vi "myRIO_BRig_Host_v0,35.vi"() -> ()   [LabVIEW 2014]
panel:
  in  "Pause":bool
  out "graph_ai1 2":dbl(graph)
  out "graph_ai0 2":dbl[](graph)
  out "graph_ai1":dbl(graph)
  out "RunTime_seconds":u16
  out "RunTime_minutes":u16
  out "BlockL_T2R_cur":u16 caption="Trials2Reward"
  out "BlockL_BTPR_cur":u16 caption="BadTrialsPostReward"
  out "BlockL_T2R_avg":dbl caption="Trials2Reward" format="%#_3g"
  out "BlockL_BTPR_avg":dbl caption="BadTrialsPostReward" format="%#_3g"
  out "BlockR_T2R_cur":u16 caption="Trials2Reward"
  out "BlockR_BTPR_cur":u16 caption="BadTrialsPostReward"
  out "BlockR_T2R_avg":dbl caption="Trials2Reward" format="%#_3g"
  out "BlockR_BTPR_avg":dbl caption="BadTrialsPostReward" format="%#_3g"
  out "error_LoadPrevSettings":errorcluster caption="error out"
  in  "LoadPrevSettings":bool
  out "graph_ai0":dbl(graph)
  in  "maxTrialsDisplayed":i32 caption="Number of Trials Displayed\n( 0 = all trials )"
  out "error_TCP":errorcluster
  in  "stop":bool
  in  "colorIn_timeout":u32(colorbox)=7468543 caption="Choice Timeout"
  in  "colorIn_wrong/cue":u32(colorbox)=16728618 caption="Wrong Choice or\nLicked During Cue"
  in  "colorIn_reward":u32(colorbox)=5898088 caption="Reward"
  in  "colorIn_unknown":u32(colorbox)=16449331 caption="Unknown Trial Status"
  out "dataOut_plot":cluster{i32[], i32[]}[](graph)
  out "iTrial":i32
  out "iBlock":i32
  # "Exp Stats"
  # "Current Block Stats"
  # "Trials 2 Reward\n\nBad Trials\nPost Reward"
  # "Left Spout    Right Spout"
  # "Run Time\n\n   minutes    seconds"
  # "Average Block Stats"
  # "Trials 2 Reward\n\nBad Trials\nPost Reward"
  # "Left Spout    Right Spout"
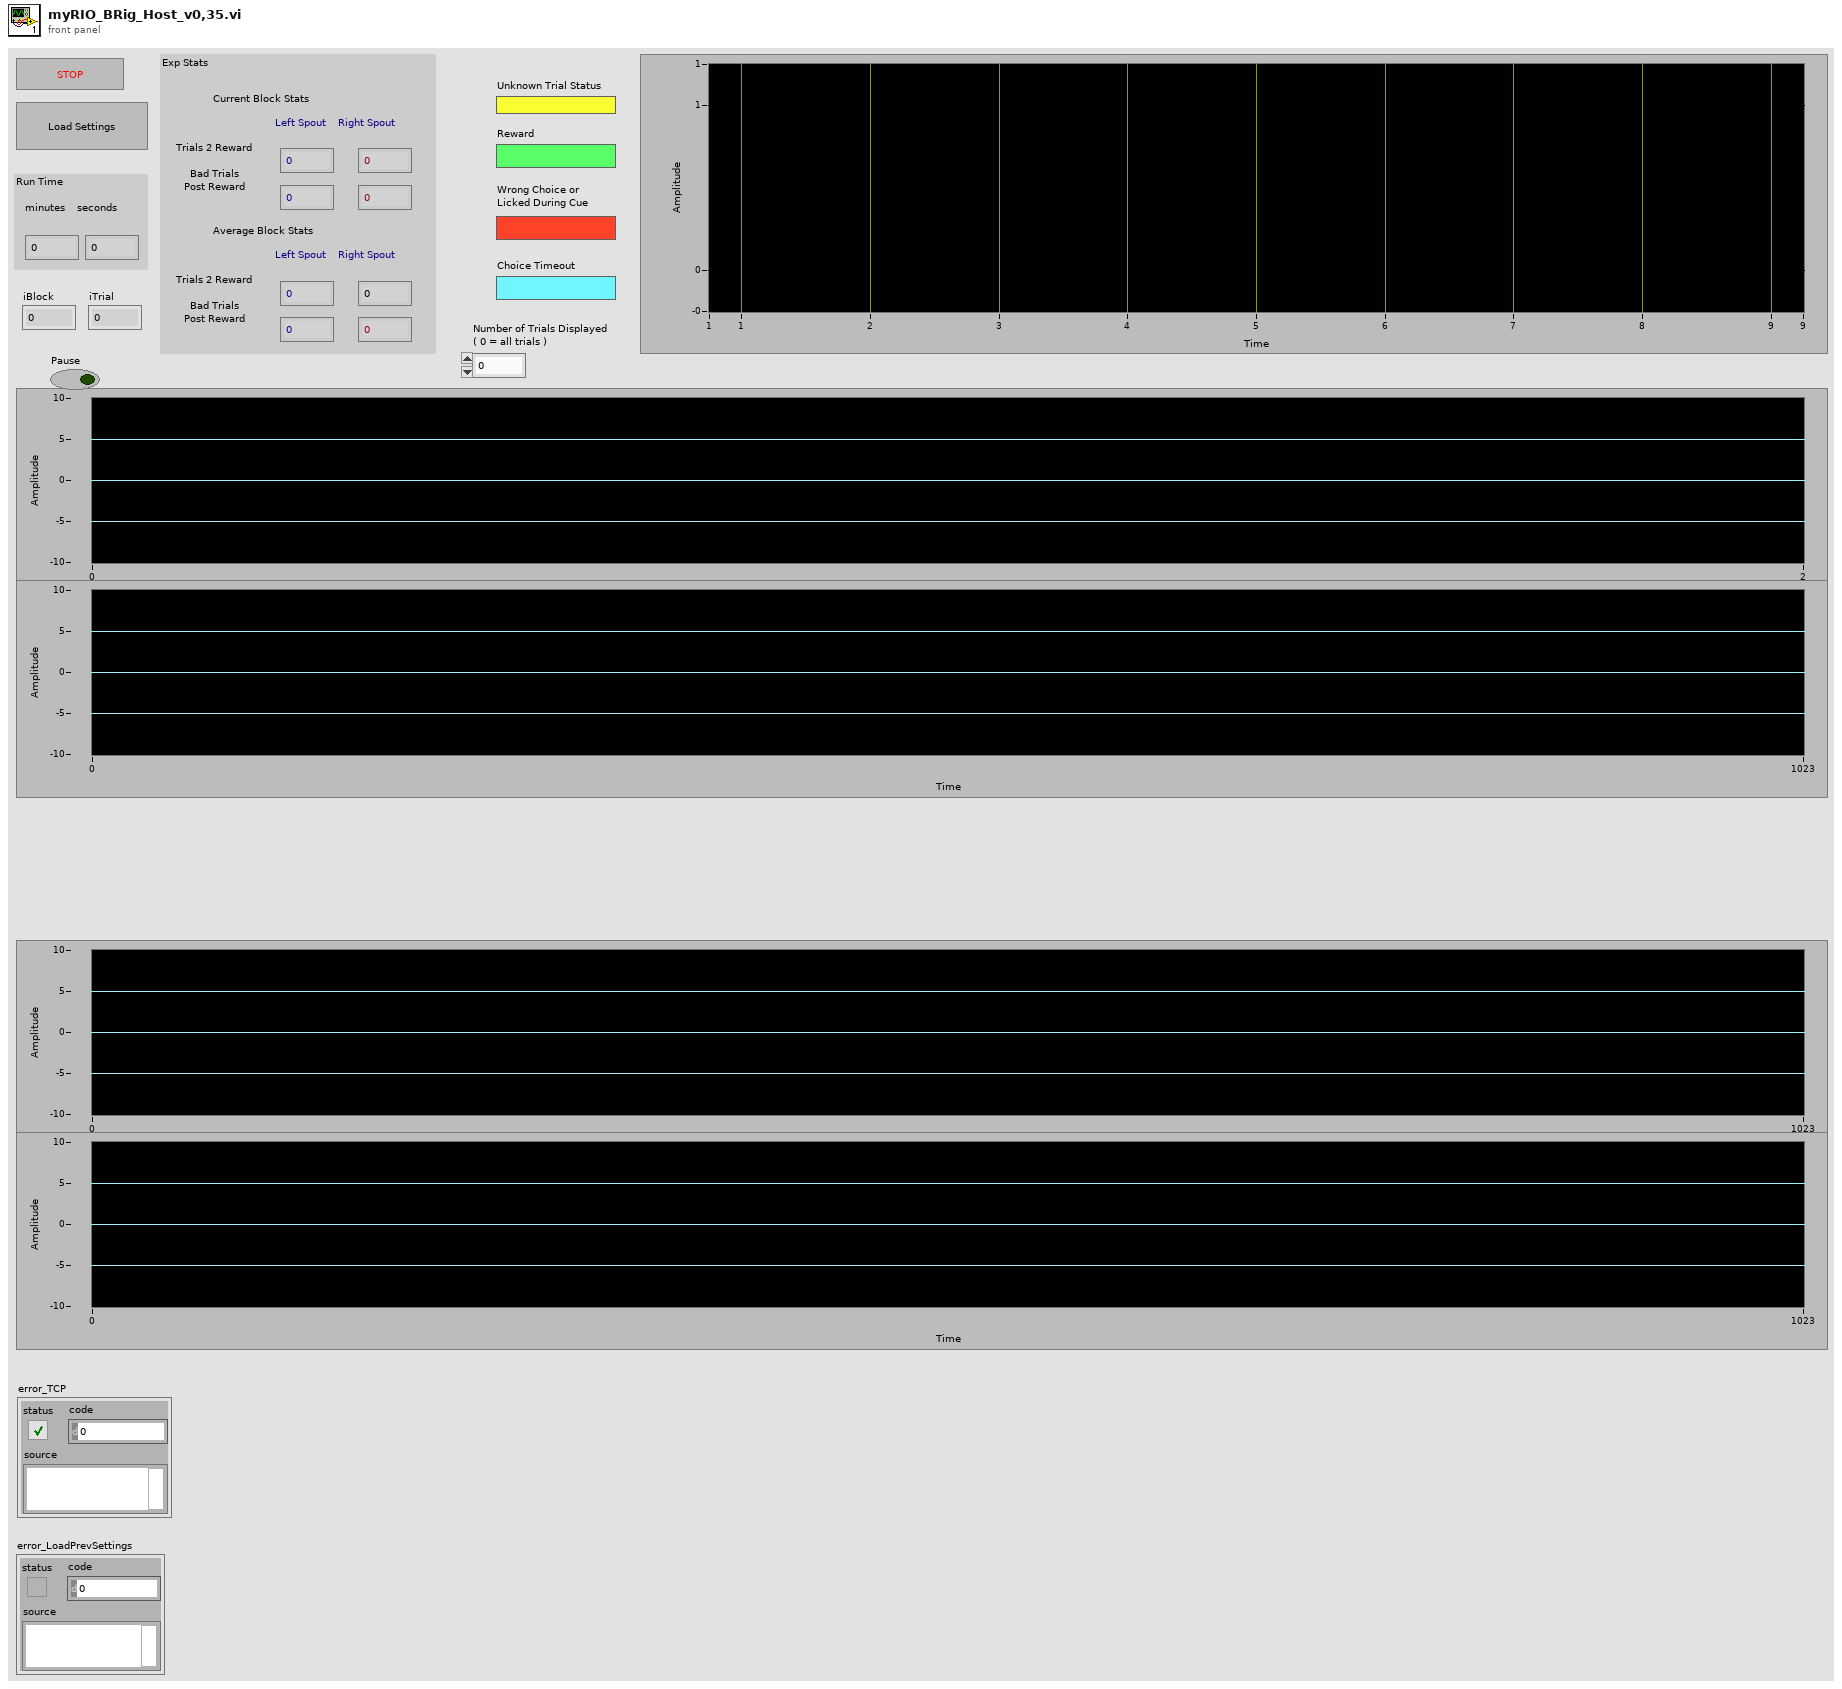
[diagram p1: front panel]
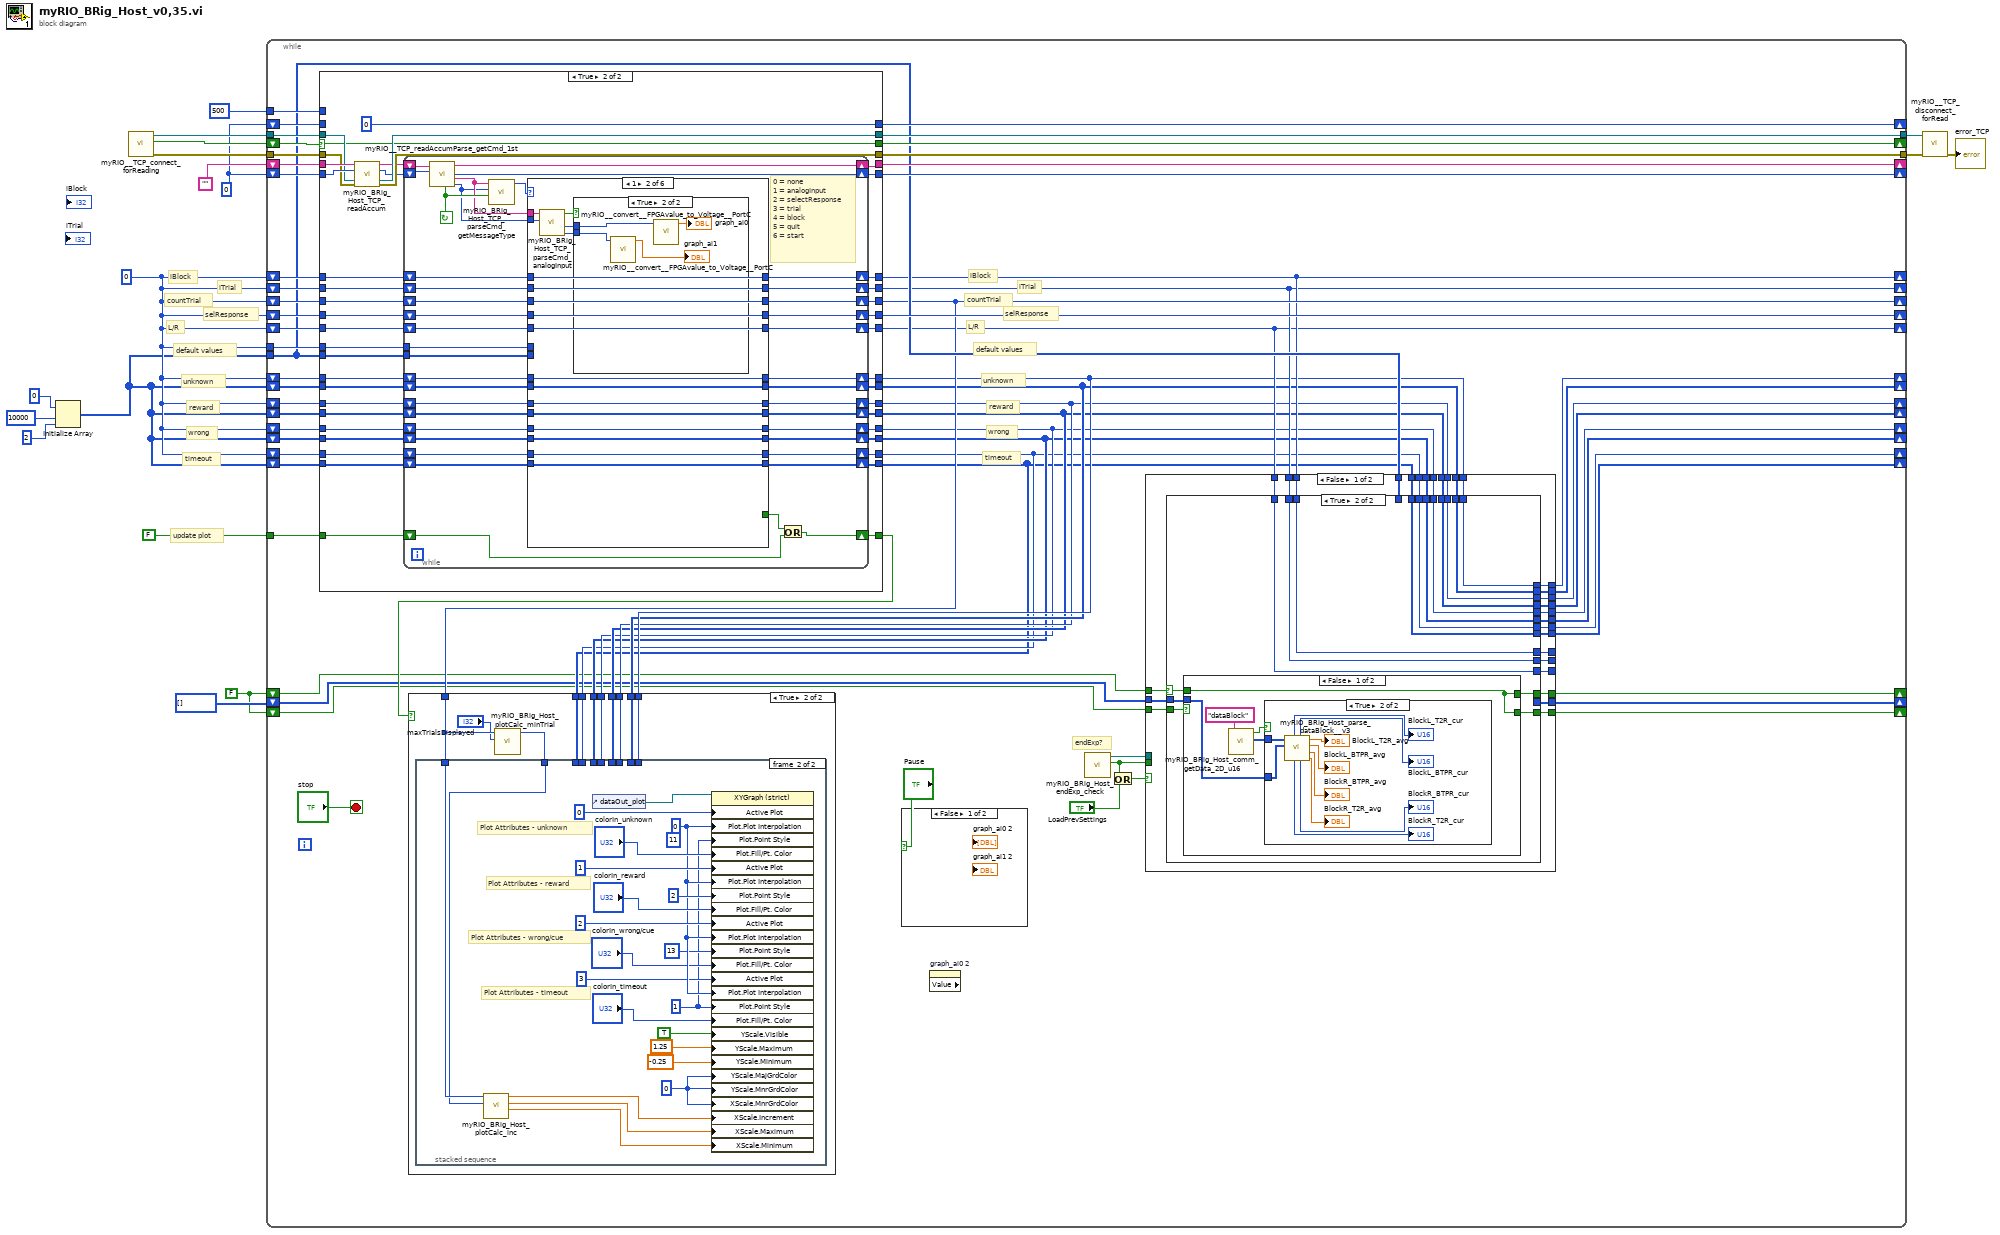
[diagram p0: block diagram]
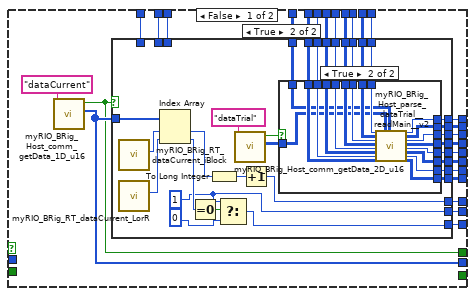
[diagram p3: hidden frame]
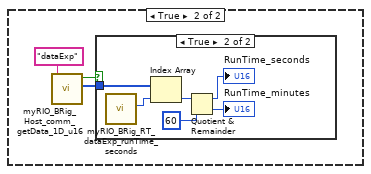
[diagram p7: hidden frame]
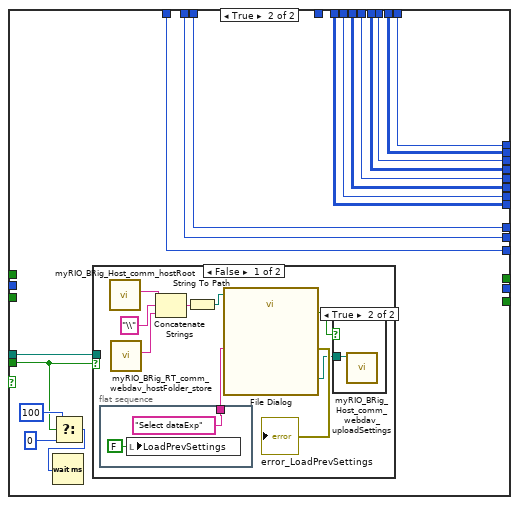
[diagram p9: hidden frame]
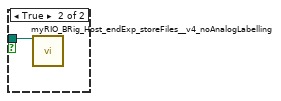
[diagram p11: hidden frame]
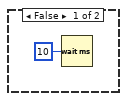
[diagram p12: hidden frame]
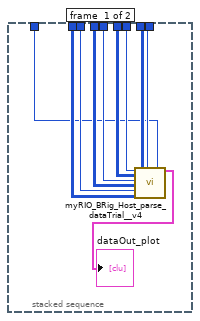
[diagram p13: hidden frame]
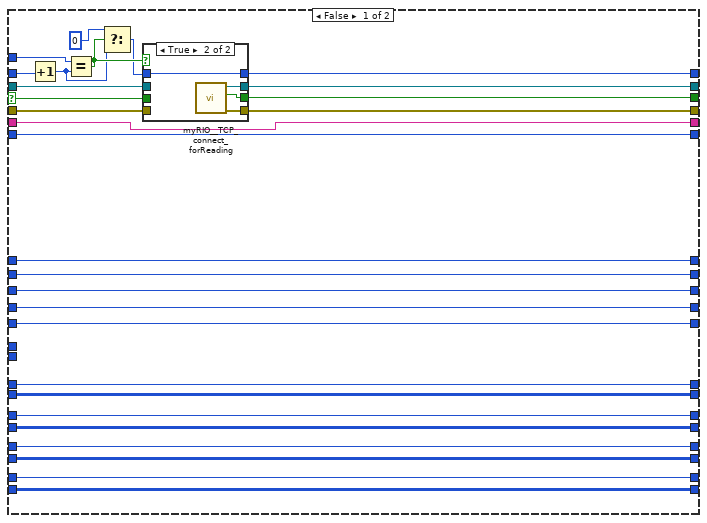
[diagram p14: hidden frame]
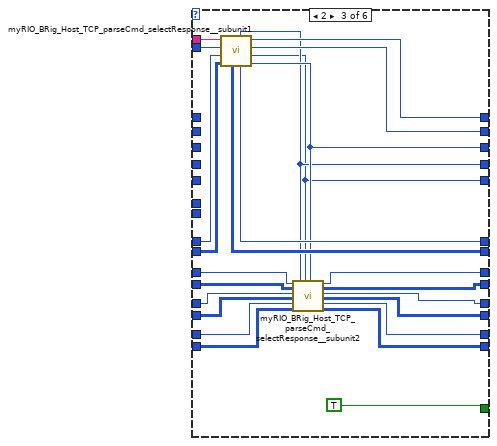
[diagram p18: hidden frame]
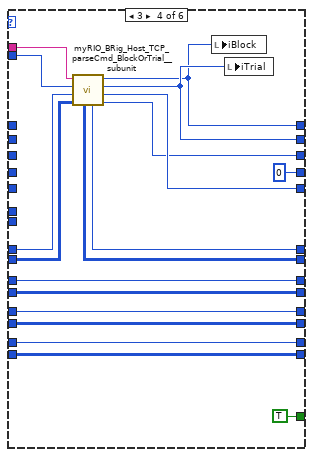
[diagram p19: hidden frame]
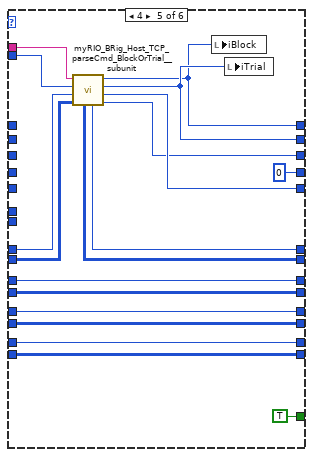
[diagram p20: hidden frame]
diagram:
  w1 = FALSE ("output_I_data")
  w4 = 0
  w13 = 0
  # "default values"
  # "update plot"
  # "timeout"
  # "wrong"
  # "reward"
  # "unknown"
  # "L/R"
  # "selResponse"
  # "countTrial"
  # "iBlock"
  # "iTrial"
  n1 = Initialize Array(0 ("element"), 10000 ("dimension size"), 2 ("dimension size")) -> (w3:i32[][])
  n2 = call "myRIO__TCP_connect_forReading.vi"() -> ("output_error"=w15:errorcluster, "output_connected"=w16:bool, "output_hTCP"=w17:refnum<k5>)  [unwired: 9 in]
  n3 = while {
    tunnel: w17 -> [w79]
    tunnel: w15 -> [w77]
    shift-right: [w70] -> _
    shift-left: w13 -> [w75]
    shift-right: [w71] -> _
    shift-left: "" -> [w76]
    shift-right: [w72] -> _
    shift-left: w16 -> [w78]
    shift-right: [w73] -> _
    shift-left: w13 -> [w80]
    tunnel: 500 ("y") -> [w74]
    shift-right: [w43] -> _
    shift-left: w4 -> [w69]
    shift-right: [w42] -> _
    shift-left: w4 -> [w68]
    shift-right: [w44] -> _
    shift-left: w4 -> [w67]
    shift-right: [w55] -> _
    shift-left: w4 -> [w66]
    shift-right: [w41] -> _
    shift-left: w4 -> [w65]
    shift-right: [w32] -> _
    shift-left: w4 -> [w64]
    shift-right: [w31] -> _
    shift-left: w3 -> [w63]
    shift-right: [w30] -> _
    shift-left: w4 -> [w62]
    shift-right: [w29] -> _
    shift-left: w3 -> [w61]
    shift-right: [w28] -> _
    shift-left: w4 -> [w60]
    shift-right: [w27] -> _
    shift-left: w3 -> [w59]
    shift-right: [w26] -> _
    shift-left: w4 -> [w58]
    shift-right: [w25] -> _
    shift-left: w3 -> [w57]
    tunnel: [w53] -> w7
    tunnel: [w52] -> w6
    tunnel: FALSE -> [w56]
    tunnel: w4 -> [w50]
    tunnel: w3 -> [w45]
    shift-right: [w24] -> _
    shift-left: u16[] [] ("output_data_1D") -> [w21]
    shift-right: [w23] -> _
    shift-left: w1 -> [w22]
    shift-right: [w19] -> _
    shift-left: w1 -> [w20]
    stop <- "stop" stop-if-true
    # "default values"
    # "timeout"
    # "wrong"
    # "reward"
    # "unknown"
    # "L/R"
    # "selResponse"
    # "countTrial"
    # "iBlock"
    # "iTrial"
    # "endExp?"
    n4 = case shown="True" w78 {
      selector: w78 -> [w340 w389]
      tunnel: w76 -> [w334 w395]
      tunnel: w75 -> [w335 w394]
      tunnel: [w334 w385] -> w71
      tunnel: [w335 w384] -> w70
      tunnel: w79 -> [w341 w393]
      tunnel: [w344 w392] -> w53
      tunnel: w77 -> [w339 w391]
      tunnel: [w343 w390] -> w52
      tunnel: [w342 w389] -> w72
      tunnel: w80 -> [w345 _]
      tunnel: [w333 0] -> w73
      tunnel: w74 -> [w332 _]
      tunnel: w69 -> [w331 w383]
      tunnel: w68 -> [w330 w382]
      tunnel: w67 -> [w329 w381]
      tunnel: w66 -> [w328 w380]
      tunnel: w65 -> [w327 w379]
      tunnel: w64 -> [w326 w378]
      tunnel: w63 -> [w325 w377]
      tunnel: w62 -> [w324 w376]
      tunnel: w61 -> [w323 w375]
      tunnel: w60 -> [w322 w374]
      tunnel: w59 -> [w321 w373]
      tunnel: w58 -> [w320 w372]
      tunnel: w57 -> [w319 w371]
      tunnel: w56 -> [_ w370]
      tunnel: [_ w369] -> w54
      tunnel: [w331 w368] -> w43
      tunnel: [w330 w367] -> w42
      tunnel: [w329 w366] -> w44
      tunnel: [w328 w365] -> w55
      tunnel: [w327 w364] -> w41
      tunnel: [w326 w363] -> w40
      tunnel: [w325 w362] -> w39
      tunnel: [w324 w361] -> w38
      tunnel: [w323 w360] -> w37
      tunnel: [w322 w359] -> w36
      tunnel: [w321 w358] -> w35
      tunnel: [w320 w357] -> w34
      tunnel: [w319 w356] -> w33
      tunnel: w50 -> [_ w355]
      tunnel: w45 -> [_ w354]
      frame False {
        n5 = Increment(x=w345) -> (x+1=w318:i32)
        n6 = Equal?(x=w332, y=w318) -> (x = y?=w338:bool)
        n7 = Select(t=0, s=w338, f=w318) -> (s? t:f=w336:i32)
        n8 = case shown="True" w338 {
          tunnel: w336 -> [w346 w350]
          tunnel: [w349 w353] -> w344
          tunnel: [w347 w352] -> w343
          tunnel: [w348 w351] -> w342
          tunnel: w341 -> [w349 _]
          tunnel: w340 -> [w348 _]
          tunnel: w339 -> [w347 _]
          tunnel: [w346 w350] -> w333
          frame False {
          }
          frame True {
            n9 = call "myRIO__TCP_connect_forReading.vi"() -> ("output_error"=w352:errorcluster, "output_connected"=w351:bool, "output_hTCP"=w353:refnum<k5>)  [unwired: 9 in]
          }
        }
      }
      frame True {
        n10 = call "myRIO_BRig_Host_TCP_readAccum.vi"("input_strAccum"=w395, "input_count"=w394, "input_handle_TCP"=w393, "input_error"=w391) -> ("output_strAccum"=w387:string, "output_count"=w386:i32, "output_handle_TCP"=w392:refnum<k5>, "output_error"=w390:errorcluster)  [unwired: 8 in]
        n11 = while {
          shift-right: [w432] -> w385
          shift-left: w387 -> [w434]
          shift-right: [w431] -> w384
          shift-left: w386 -> [w433]
          shift-right: [w423] -> w368
          shift-left: w383 -> [w426]
          shift-right: [w422] -> w367
          shift-left: w382 -> [w425]
          shift-right: [w421] -> w366
          shift-left: w381 -> [w424]
          shift-right: [w419] -> w365
          shift-left: w380 -> [w420]
          shift-right: [w417] -> w364
          shift-left: w379 -> [w418]
          shift-right: [w415] -> w363
          shift-left: w378 -> [w416]
          shift-right: [w413] -> w362
          shift-left: w377 -> [w414]
          shift-right: [w406] -> w361
          shift-left: w376 -> [w412]
          shift-right: [w405] -> w360
          shift-left: w375 -> [w411]
          shift-right: [w404] -> w359
          shift-left: w374 -> [w410]
          shift-right: [w403] -> w358
          shift-left: w373 -> [w409]
          shift-right: [w401] -> w356
          shift-left: w371 -> [w407]
          shift-right: [w402] -> w357
          shift-left: w372 -> [w408]
          shift-right: [w399] -> w369
          shift-left: w370 -> [w396]
          tunnel: w355 -> [w398]
          tunnel: w354 -> [w397]
          stop <- w430 continue-if-true
          # "0 = none\n1 = analogInput\n2 = selectResponse\n3 = trial\n4 = block\n5 = quit\n6 = start"
          n12 = call "myRIO__TCP_readAccumParse_getCmd_1st.vi"("input_count"=w433, "input_strAccum"=w434) -> ("output_countCmd"=w428:i32, "output_strCmd"=w429:string, "output_count"=w431:i32, "output_strAccum"=w432:string, "output_haveCmd"=w430:bool)  [unwired: 5 in]
          n13 = call "myRIO_BRig_Host_TCP_parseCmd_getMessageType.vi"("input_haveCmd"=w430, "input_countCmd"=w428, "input_strCmd"=w429) -> ("output_messageType"=w427:u8)  [unwired: 8 in]
          n14 = case shown="1" w427 {
            tunnel: w429 -> [_ w452 w493 w510 w528 w563]
            tunnel: w428 -> [_ w451 w492 w509 w527 _]
            tunnel: w426 -> [w447 w465 _ _ _ w558]
            tunnel: w425 -> [w446 w464 _ _ _ w556]
            tunnel: w424 -> [w445 w463 _ _ _ w555]
            tunnel: [w447 w465 w487 w495 w513 w557] -> w423
            tunnel: [w446 w464 w486 w496 w514 w552] -> w422
            tunnel: [w445 w463 w485 w503 w521 w551] -> w421
            tunnel: w420 -> [w444 w462 _ _ _ w554]
            tunnel: [w444 w462 w484 0 ("output_iTrial_num") 0 ("output_iTrial_num") w550] -> w419
            tunnel: w418 -> [w443 w461 _ _ _ w553]
            tunnel: [w443 w461 w483 w504 w522 w549] -> w417
            tunnel: w416 -> [w442 w460 w491 w508 w526 w548]
            tunnel: [w442 w460 w489 w506 w524 w540] -> w415
            tunnel: w414 -> [w441 w459 w490 w507 w525 w547]
            tunnel: [w441 w459 w488 w505 w523 w539] -> w413
            tunnel: w412 -> [w440 w458 w482 w502 w520 w546]
            tunnel: w411 -> [w439 w457 w481 w501 w519 w545]
            tunnel: w410 -> [w438 w456 w480 w500 w518 w544]
            tunnel: w409 -> [w437 w455 w479 w499 w517 w543]
            tunnel: w408 -> [w436 w454 w478 w498 w516 w542]
            tunnel: w407 -> [w435 w453 w477 w497 w515 w541]
            tunnel: [w440 w458 w476 w502 w520 w538] -> w406
            tunnel: [w439 w457 w475 w501 w519 w537] -> w405
            tunnel: [w438 w456 w474 w500 w518 w536] -> w404
            tunnel: [w437 w455 w473 w499 w517 w535] -> w403
            tunnel: [w436 w454 w472 w498 w516 w534] -> w402
            tunnel: [w435 w453 w471 w497 w515 w533] -> w401
            tunnel: [_ _ TRUE TRUE TRUE w530] -> w400
            tunnel: w398 -> [_ _ _ _ _ w532]
            tunnel: w397 -> [_ _ _ _ _ w531]
            frame 0, Default {
            }
            frame 1 {
              n15 = call "myRIO_BRig_Host_TCP_parseCmd_analogInput.vi"("input_countCmd"=w451, "input_strCmd"=w452) -> ("output_ai1"=w448:i32, "output_ai0"=w449:i32, "output_haveAnalogInput"=w450:bool)  [unwired: 7 in]
              n16 = case shown="True" w450 {
                tunnel: w449 -> [_ w469]
                tunnel: w448 -> [_ w467]
                frame False {
                }
                frame True {
                  n17 = call "myRIO__convert__FPGAvalue_to_Voltage__PortC.vi"("input_FPGAvalue_PortC"=w467) -> ("output_voltage"=→"graph_ai1":dbl)  [unwired: 10 in]
                  n18 = call "myRIO__convert__FPGAvalue_to_Voltage__PortC.vi"("input_FPGAvalue_PortC"=w469) -> ("output_voltage"=→"graph_ai0":dbl)  [unwired: 10 in]
                }
              }
            }
            frame 2 {
              n19 = call "myRIO_BRig_Host_TCP_parseCmd_selectResponse__subunit1.vi"("input_arrayUnknown"=w490, "input_idxUnknown"=w491, "input_countCmd"=w492, "input_strCmd"=w493) -> ("output_countTrial"=w485:i32, "output_L/R"=w483:i32, "output_iTrial"=w486:i32, "output_iBlock"=w487:i32, "output_idxUnknown"=w489:i32, "output_response"=w484:i32, "output_arrayUnknown"=w488:i32[][])  [unwired: 1 in]
              n20 = call "myRIO_BRig_Host_TCP_parseCmd_selectResponse__subunit2.vi"("input_idxReward"=w482, "input_arrayReward"=w481, "input_idxWrong"=w480, "input_arrayWrong"=w479, "input_idxTimeout"=w478, "input_arrayTimeout"=w477, "input_response"=w484, "input_L/R"=w483, "input_countTrial"=w485) -> ("output_idxReward"=w476:i32, "output_arrayReward"=w475:i32[][], "output_idxWrong"=w474:i32, "output_arrayWrong"=w473:i32[][], "output_idxTimeout"=w472:i32, "output_arrayTimeout"=w471:i32[][])  [unwired: 5 in]
            }
            frame 3 {
              n21 = call "myRIO_BRig_Host_TCP_parseCmd_BlockOrTrial__subunit.vi"("input_arrayUnknown"=w507, "input_idxUnknown"=w508, "input_countCmd"=w509, "input_strCmd"=w510) -> ("output_countTrial"=w503:i32, "output_L/R"=w504:i32, "output_iTrial"=w496:i32, "output_iBlock"=w495:i32, "output_idxUnknown"=w506:i32, "output_arrayUnknown"=w505:i32[][])  [unwired: 2 in]
              n22 = local write "iBlock"(w495) -> ()
              n23 = local write "iTrial"(w496) -> ()
            }
            frame 4 {
              n24 = call "myRIO_BRig_Host_TCP_parseCmd_BlockOrTrial__subunit.vi"("input_arrayUnknown"=w525, "input_idxUnknown"=w526, "input_countCmd"=w527, "input_strCmd"=w528) -> ("output_countTrial"=w521:i32, "output_L/R"=w522:i32, "output_iTrial"=w514:i32, "output_iBlock"=w513:i32, "output_idxUnknown"=w524:i32, "output_arrayUnknown"=w523:i32[][])  [unwired: 2 in]
              n25 = local write "iBlock"(w513) -> ()
              n26 = local write "iTrial"(w514) -> ()
            }
            frame 6 {
              n27 = String Subset(string=w563, offset (0)=2, length (rest)=1 ("length (rest)")) -> (substring=w560:string)
              n28 = Equal?(x=w560, y="e") -> (x = y?=w530:bool)
              n29 = case shown="True" w530 {
                tunnel: w558 -> [w576 _]
                tunnel: [w576 w578] -> w557
                tunnel: w556 -> [w575 _]
                tunnel: w555 -> [w574 _]
                tunnel: w554 -> [w573 _]
                tunnel: w553 -> [w572 _]
                tunnel: [w575 w578] -> w552
                tunnel: [w574 w578] -> w551
                tunnel: [w573 w578] -> w550
                tunnel: [w572 w578] -> w549
                tunnel: w548 -> [w571 _]
                tunnel: w547 -> [w570 _]
                tunnel: w546 -> [w569 _]
                tunnel: w545 -> [w568 _]
                tunnel: w544 -> [w567 _]
                tunnel: w543 -> [w566 _]
                tunnel: w542 -> [w565 _]
                tunnel: w541 -> [w564 _]
                tunnel: [w571 w578] -> w540
                tunnel: [w570 w577] -> w539
                tunnel: [w569 w578] -> w538
                tunnel: [w568 w577] -> w537
                tunnel: [w567 w578] -> w536
                tunnel: [w566 w577] -> w535
                tunnel: [w565 w578] -> w534
                tunnel: [w564 w577] -> w533
                tunnel: w532 -> [_ w578]
                tunnel: w531 -> [_ w577]
                frame False {
                }
                frame True {
                }
              }
            }
          }
          n30 = Or(x=w400, y=w396) -> (x .or. y?=w399:bool)
        }
      }
    }
    n31 = case shown="True" w54 {
      tunnel: w33 -> [_ w285]
      tunnel: w34 -> [_ w284]
      tunnel: w35 -> [_ w283]
      tunnel: w36 -> [_ w282]
      tunnel: w37 -> [_ w281]
      tunnel: w38 -> [_ w280]
      tunnel: w39 -> [_ w279]
      tunnel: w40 -> [_ w278]
      tunnel: w44 -> [_ w277]
      frame False {
        n32 = Wait (ms)(milliseconds to wait=u32 10) -> ()  [unwired: 1 out]
      }
      frame True {
        n33 = call "myRIO_BRig_Host_plotCalc_minTrial.vi"("input_maxTrialsDisplayed"="maxTrialsDisplayed", "input_countTrial"=w277) -> ("output_minTrial"=w275:i32)  [unwired: 9 in]
        n34 = stacked-sequence {
          tunnel: w285 -> [w295 _]
          tunnel: w284 -> [w294 _]
          tunnel: w283 -> [w293 _]
          tunnel: w282 -> [w292 _]
          tunnel: w281 -> [w291 _]
          tunnel: w280 -> [w290 _]
          tunnel: w279 -> [w289 _]
          tunnel: w278 -> [w288 _]
          tunnel: w275 -> [w286 w299]
          tunnel: w277 -> [_ w300]
          frame #0 {
            n35 = call "myRIO_BRig_Host_parse_dataTrial__v4.vi"("input_idxReward"=w290, "input_arrayReward"=w291, "input_idxWrong"=w292, "input_arrayWrong"=w293, "input_idxTimeout"=w294, "input_arrayTimeout"=w295, "input_arrayUnknown"=w289, "input_idxUnknown"=w288, "input_minTrial"=w286) -> ("output_plotData"=→"dataOut_plot":cluster{i32[], i32[]}[])  [unwired: 10 in]
          }
          frame #1 {
            w302 = u32 0 ("Y Scale.Grid Colors:Major Color")
            w301 = u8 1 ("Plot.Point Style")
            (unwired) u8 11 ("Plot.Point Style")
            w311 = u8 0 ("Plot.Plot Interpolation")
            # "Plot Attributes - timeout"
            # "Plot Attributes - wrong/cue"
            # "Plot Attributes - reward"
            # "Plot Attributes - unknown"
            n36 = call "myRIO_BRig_Host_plotCalc_inc.vi"("input_minTrial"=w299, "input_countTrial"=w300) -> ("output_min"=w296:dbl, "output_max"=w297:dbl, "output_inc"=w298:dbl)  [unwired: 7 in]
            n37 = control-ref of="dataOut_plot"() -> (w306:refnum<vi>)
            n38 = property on="Property Node" class="XYGraph (strict)"(reference=w306, "Active Plot"=u32 0, "Plot.Plot Interpolation"=w311, "Plot.Point Style"=w301, "Plot.Fill/Pt. Color"="colorIn_unknown", "Active Plot"=u32 1, "Plot.Plot Interpolation"=w311, "Plot.Point Style"=u8 2, "Plot.Fill/Pt. Color"="colorIn_reward", "Active Plot"=u32 2, "Plot.Plot Interpolation"=w311, "Plot.Point Style"=u8 13, "Plot.Fill/Pt. Color"="colorIn_wrong/cue", "Active Plot"=u32 3, "Plot.Plot Interpolation"=w311, "Plot.Point Style"=w301, "Plot.Fill/Pt. Color"="colorIn_timeout", "YScale.Visible"=TRUE ("Y Scale.Visible"), "YScale.Maximum"=1.25 ("Y Scale.Range:Maximum"), "YScale.Minimum"=-0.25 ("Y Scale.Range:Minimum"), "YScale.MajGrdColor"=w302, "YScale.MnrGrdColor"=w302, "XScale.MnrGrdColor"=w302, "XScale.Increment"=w298, "XScale.Maximum"=w297, "XScale.Minimum"=w296) -> ()  [unwired: 1 in, 2 out]
          }
        }
      }
    }
    n39 = case shown="False" "Pause" {
      frame False {
      }
      frame True {
      }
    }
    n40 = property on="graph_ai0 2" class="WFChart (strict)" props=["Value"]() -> ()  [unwired: 2 in, 3 out]
    n41 = call "myRIO_BRig_Host_endExp_check.vi"() -> ("output_IendExp"=w47:bool, "output_filePath_expExp"=w46:path)  [unwired: 10 in]
    n42 = Or(x=w47, y="LoadPrevSettings") -> (x .or. y?=w48:bool)
    n43 = case shown="False" w48 {
      tunnel: w47 -> [_ w257]
      tunnel: w46 -> [_ w256]
      tunnel: [w110 w255] -> w32
      tunnel: [w109 w254] -> w31
      tunnel: [w108 w253] -> w30
      tunnel: [w107 w252] -> w29
      tunnel: [w106 w251] -> w28
      tunnel: [w105 w250] -> w27
      tunnel: [w104 w249] -> w26
      tunnel: [w103 w248] -> w25
      tunnel: w40 -> [w102 w255]
      tunnel: w39 -> [w101 w254]
      tunnel: w38 -> [w100 w253]
      tunnel: w37 -> [w99 w252]
      tunnel: w36 -> [w98 w251]
      tunnel: w35 -> [w97 w250]
      tunnel: w34 -> [w96 w249]
      tunnel: w33 -> [w95 w248]
      tunnel: w45 -> [w94 _]
      tunnel: [w93 w245] -> _
      tunnel: [w92 w246] -> _
      tunnel: [w91 w247] -> _
      tunnel: w43 -> [w90 w247]
      tunnel: w42 -> [w89 w246]
      tunnel: w41 -> [w88 w245]
      tunnel: [w87 _] -> w24
      tunnel: [w86 _] -> w23
      tunnel: w22 -> [w85 _]
      tunnel: w21 -> [w84 _]
      tunnel: w20 -> [w83 _]
      tunnel: [w82 _] -> w19
      frame False {
        n44 = case shown="True" w85 {
          selector: w85 -> [_ w206]
          tunnel: [w135 w220] -> w110
          tunnel: [w134 w219] -> w109
          tunnel: [w133 w218] -> w108
          tunnel: [w132 w217] -> w107
          tunnel: [w131 w216] -> w106
          tunnel: [w130 w215] -> w105
          tunnel: [w129 w214] -> w104
          tunnel: [w128 w213] -> w103
          tunnel: w102 -> [w127 w220]
          tunnel: w101 -> [w126 w219]
          tunnel: w100 -> [w125 w218]
          tunnel: w99 -> [w124 w217]
          tunnel: w98 -> [w123 w216]
          tunnel: w97 -> [w122 w215]
          tunnel: w96 -> [w121 w214]
          tunnel: w95 -> [w120 w213]
          tunnel: w94 -> [w119 _]
          tunnel: [w118 w210] -> w93
          tunnel: [w117 w211] -> w92
          tunnel: [w116 w212] -> w91
          tunnel: w90 -> [w115 w212]
          tunnel: w89 -> [w114 w211]
          tunnel: w88 -> [w113 w210]
          tunnel: [w112 _] -> w87
          tunnel: [w111 w207] -> w86
          tunnel: w84 -> [_ w209]
          tunnel: w83 -> [_ w208]
          tunnel: [_ w205] -> w82
          frame False {
            n45 = call "myRIO_BRig_Host_comm_getData_1D_u16.vi"("input_fileName"="dataCurrent") -> ("output_data_1D"=w112:u16[], "output_I_data"=w111:bool)  [unwired: 9 in]
            n46 = case shown="True" w111 {
              tunnel: w112 -> [_ w178]
              tunnel: [w147 w173] -> w135
              tunnel: [w146 w172] -> w134
              tunnel: [w145 w171] -> w133
              tunnel: [w144 w170] -> w132
              tunnel: [w143 w169] -> w131
              tunnel: [w142 w168] -> w130
              tunnel: [w141 w167] -> w129
              tunnel: [w140 w166] -> w128
              tunnel: w127 -> [w147 w165]
              tunnel: w126 -> [w146 w164]
              tunnel: w125 -> [w145 w163]
              tunnel: w124 -> [w144 w162]
              tunnel: w123 -> [w143 w161]
              tunnel: w122 -> [w142 w160]
              tunnel: w121 -> [w141 w159]
              tunnel: w120 -> [w140 w158]
              tunnel: w119 -> [_ w157]
              tunnel: [w137 w153] -> w118
              tunnel: [w138 w152] -> w117
              tunnel: [w139 w148] -> w116
              tunnel: w115 -> [w139 _]
              tunnel: w114 -> [w138 _]
              tunnel: w113 -> [w137 _]
              frame False {
              }
              frame True {
                w152 = 1
                n47 = call "myRIO_BRig_RT_dataCurrent_iBlock.vi"() -> ("output_iBlock"=w151:i32)  [unwired: 11 in]
                n48 = call "myRIO_BRig_RT_dataCurrent_LorR.vi"() -> ("output_LorR"=w174:i32)  [unwired: 11 in]
                n49 = Index Array(array=w178, index #1=w151, index #2=w174) -> (element #1=w150:u16, element #2=w156:u16)
                n50 = Equal To 0?(x=w156) -> (x = 0?=w155:bool)
                n51 = To Long Integer(number=w150) -> (32bit integer=w149:i32)
                n52 = Select(t=w152, s=w155, f=0) -> (s? t:f=w153:i32)
                n53 = call "myRIO_BRig_Host_comm_getData_2D_u16.vi"("input_fileName"="dataTrial") -> ("output_data_2D"=w175:u16[][], "output_I_data"=w176:bool)  [unwired: 9 in]
                n54 = Increment(x=w149) -> (x+1=w148:i32)
                n55 = case shown="True" w176 {
                  tunnel: w175 -> [_ w196]
                  tunnel: [w184 w192] -> w171
                  tunnel: [w183 w191] -> w170
                  tunnel: [w185 w193] -> w172
                  tunnel: [w186 w194] -> w173
                  tunnel: [w182 w190] -> w169
                  tunnel: [w181 w189] -> w168
                  tunnel: [w180 w188] -> w167
                  tunnel: [w179 w187] -> w166
                  tunnel: w157 -> [_ w195]
                  tunnel: w165 -> [w186 w204]
                  tunnel: w164 -> [w185 w203]
                  tunnel: w163 -> [w184 w202]
                  tunnel: w162 -> [w183 w201]
                  tunnel: w161 -> [w182 w200]
                  tunnel: w160 -> [w181 w199]
                  tunnel: w159 -> [w180 w198]
                  tunnel: w158 -> [w179 w197]
                  frame False {
                  }
                  frame True {
                    n56 = call "myRIO_BRig_Host_parse_dataTrial__readMain__v2.vi"("input_idxUnknown"=w204, "input_arrayUnknown"=w203, "input_idxReward"=w202, "input_arrayReward"=w201, "input_idxWrong"=w200, "input_arrayWrong"=w199, "input_idxTimeout"=w198, "input_arrayTimeout"=w197, "arrayIn_dataTrial"=w196, "arrayIn_empty"=w195) -> ("output_idxUnknown"=w194:i32, "output_arrayUnknown"=w193:i32[][], "output_idxReward"=w192:i32, "output_arrayReward"=w191:i32[][], "output_idxWrong"=w190:i32, "output_arrayWrong"=w189:i32[][], "output_idxTimeout"=w188:i32, "output_arrayTimeout"=w187:i32[][])  [unwired: 10 in]
                  }
                }
              }
            }
          }
          frame True {
            n57 = case shown="False" w208 {
              tunnel: w209 -> [w222 _]
              tunnel: [w221 _] -> w207
              tunnel: w206 -> [w221 _]
              tunnel: [w221 _] -> w205
              frame False {
                n58 = call "myRIO_BRig_Host_comm_getData_2D_u16.vi"("input_fileName"="dataBlock") -> ("output_data_2D"=w223:u16[][], "output_I_data"=w224:bool)  [unwired: 9 in]
                n59 = case shown="True" w224 {
                  tunnel: w223 -> [_ w227]
                  tunnel: w222 -> [_ w226]
                  frame False {
                  }
                  frame True {
                    n60 = call "myRIO_BRig_Host_parse_dataBlock__v3.vi"("input_dataCurrent"=w226, "input_dataBlock"=w227) -> ("BlockR_T2R_avg"=→"BlockR_T2R_avg":dbl, "BlockR_BTPR_avg"=→"BlockR_BTPR_avg":dbl, "BlockL_BTPR_avg"=→"BlockL_BTPR_avg":dbl, "BlockL_T2R_avg"=→"BlockL_T2R_avg":dbl, "BlockR_BTPR_cur"=→"BlockR_BTPR_cur":u16, "BlockL_BTPR_cur"=→"BlockL_BTPR_cur":u16, "BlockR_T2R_cur"=→"BlockR_T2R_cur":u16, "BlockL_T2R_cur"=→"BlockL_T2R_cur":u16)  [unwired: 2 in]
                  }
                }
              }
              frame True {
                n61 = call "myRIO_BRig_Host_comm_getData_1D_u16.vi"("input_fileName"="dataExp") -> ("output_data_1D"=w238:u16[], "output_I_data"=w237:bool)  [unwired: 9 in]
                n62 = case shown="True" w237 {
                  tunnel: w238 -> [_ w244]
                  frame False {
                  }
                  frame True {
                    n63 = call "myRIO_BRig_RT_dataExp_runTime_seconds.vi"() -> ("output_RunTime_minutes"=w243:i32)  [unwired: 11 in]
                    n64 = Index Array(array=w244, index=w243) -> (element=w242:u16)
                    n65 = Quotient & Remainder(x=w242, y=u16 60) -> (x-y*floor(x/y)=→"RunTime_seconds":u16, floor(x/y)=→"RunTime_minutes":u16)
                  }
                }
              }
            }
          }
        }
      }
      frame True {
        n66 = Select(t=u32 100 ("milliseconds to wait"), s=w257, f=u32 0 ("milliseconds to wait")) -> (s? t:f=w259:u32)
        n67 = Wait (ms)(milliseconds to wait=w259) -> ()  [unwired: 1 out]
        n68 = case shown="False" w257 {
          tunnel: w256 -> [_ w273]
          frame False {
            n69 = flat-sequence {
              tunnel: ["Select dataExp" ("prompt")] -> w264
              frame #0 {
                n70 = local write "LoadPrevSettings"(FALSE ("LoadPrevSettings")) -> ()
              }
            }
            n71 = call "myRIO_BRig_Host_comm_hostRoot.vi"() -> ("output_hostRoot"=w266:string)  [unwired: 11 in]
            n72 = call "myRIO_BRig_RT_comm_webdav_hostFolder_store.vi"() -> ("output_HostFolder"=w268:string)  [unwired: 11 in]
            n73 = Concatenate Strings(w266, "\\" ("string"), w268) -> (w269:string)
            n74 = String To Path(string=w269) -> (path=w265:path)
            n75 = call "File Dialog"("start path"=w265, "prompt"=w264) -> ("selected path"=w261:path, "exists"=w262:bool, "error out"=→"error_LoadPrevSettings":errorcluster)  [unwired: 10 in, 1 out]
            n76 = case shown="True" w262 {
              tunnel: w261 -> [_ w270]
              frame False {
              }
              frame True {
                n77 = call "myRIO_BRig_Host_comm_webdav_uploadSettings.vi"("input_filePath"=w270) -> ()  [unwired: 11 in]
              }
            }
          }
          frame True {
            n78 = call "myRIO_BRig_Host_endExp_storeFiles__v4_noAnalogLabelling.vi"("input_filePath"=w273) -> ()  [unwired: 15 in]
          }
        }
      }
    }
  }
  n79 = call "myRIO__TCP_disconnect_forRead.vi"("input_error"=w6, "input_hTCP"=w7) -> ("output_error"=→"error_TCP":errorcluster)  [unwired: 9 in]
